vi "EmsaInitialize.vi"(8 "error in (no error)":errorcluster) -> (0 "error out":errorcluster, 3 "Qbus out":refnum<class "Qbus.lvclass">)   [LabVIEW 2017]
uses:
  <vilib>/addons/Qbus/Qbus.lvclass
  <vilib>/addons/TraceLogger/TraceLogger.lvlib
  <vilib>/addons/SystemInfoProcess/SystemInfoProcess.lvlib
  <vilib>/addons/InsightCM/Utilities/GlobalConfiguration/GlobalConfiguration.lvlib
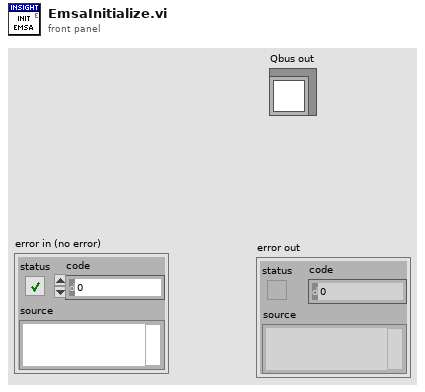
[diagram p1: front panel]
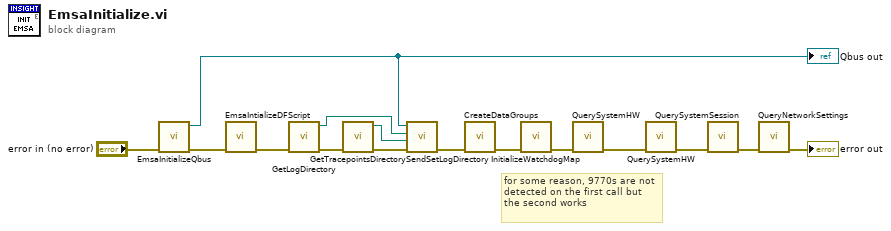
[diagram p0: block diagram]
diagram:
  # "for some reason, 9770s are not detected on the first call but the second works"
  n1 = call <vilib>:"EmsaInitializeQbus.vi"("error in (no error)"="error in (no error)") -> ("error out"=w12:errorcluster, "Qbus out"=w13:refnum<class "Qbus.lvclass">)  [unwired: 9 in]
  "Qbus out" <- w13
  n2 = call <vilib>:"EmsaIntializeDFScript.vi"("error in (no error)"=w12) -> ("error out"=w3:errorcluster)  [unwired: 10 in]
  n3 = call <vilib>:"GetLogDirectory.vi"("error in (no error)"=w3) -> ("error out"=w6:errorcluster, "log dir"=w9:path)  [unwired: 9 in]
  n4 = call <vilib>:"GetTracepointsDirectory.vi"("error in (no error)"=w6) -> ("error out"=w4:errorcluster, "application directory"=w5:path)  [unwired: 9 in]
  n5 = call <vilib>:"SendSetLogDirectory.vi"("error in (no error)"=w4, "tracpoint directory"=w5, "log directory"=w9, "qbus in"=w13) -> ("error out"=w14:errorcluster)  [unwired: 6 in, 1 out]
  n6 = call <vilib>:"CreateDataGroups.vi"("error in (no error)"=w14) -> ("error out"=w8:errorcluster)  [unwired: 10 in]
  n7 = call <vilib>:"InitializeWatchdogMap.vi"("error in (no error)"=w8) -> ("error out"=w7:errorcluster)  [unwired: 10 in]
  n8 = call <vilib>:"QuerySystemHW.vi"("error in (no error)"=w7) -> ("error out"=w2:errorcluster)  [unwired: 10 in]
  n9 = call <vilib>:"QuerySystemHW.vi"("error in (no error)"=w2) -> ("error out"=w1:errorcluster)  [unwired: 10 in]
  n10 = call <vilib>:"QuerySystemSession.vi"("error in (no error)"=w1) -> ("error out"=w11:errorcluster)  [unwired: 10 in]
  n11 = call <vilib>:"QueryNetworkSettings.vi"("error in (no error)"=w11) -> ("error out"=→"error out":errorcluster)  [unwired: 10 in]
